vi "Write Data.vi"(8 "error in (no error)":errorcluster, 9 "Publication Time":timestamp, 10 "Value":variant, 11 "TerminalVisibilityBinding In":refnum<class "TerminalVisibilityBinding.lvclass">) -> (0 "error out":errorcluster, 3 "TerminalVisibilityBinding Out":refnum<class "TerminalVisibilityBinding.lvclass">)   [LabVIEW 2020, in "TerminalVisibilityBinding.lvclass"]
doc: "<License>\nCopyright © 2017 Composed Systems, LLC | All rights reserved\nwww.composed.io\n\nAuthor: Ethan Stern <ethan.stern@composed.io>\n\nThis software is provided \"AS IS\" WITHOUT WARRANTIES, either express or implied, AND IS FOR EDUCATIONAL PURPOSES ONLY.\n</License>"
uses:
  <vilib>/gpm_packages/@cs/transport/Source/Concrete/TerminalVisibilityBinding/TerminalVisibilityBinding.lvclass
  C:/Program Files/National Instruments/LabVIEW 2020/vi.lib/gpm_packages/@cs/transport/Source/Concrete/TerminalPropertyBinding/TerminalPropertyBinding.lvclass
  <vilib>/gpm_packages/@cs/transport/Source/Concrete/TerminalPropertyBinding/TerminalPropertyBinding.lvclass/TerminalPropertyBinding.ctl
  <vilib>/gpm_packages/@cs/transport/Source/Concrete/TerminalVisibilityBinding/TerminalVisibilityBinding.lvclass/TerminalVisibilityBinding.ctl
  <vilib>/Utility/error.llb/Error Cluster From Error Code.vi
  <vilib>/ErrorRing/Error Ring.xnode
  <vilib>/gpm_packages/@cs/transport/Source/Concrete/TerminalPropertyBinding/TerminalPropertyBinding.lvclass
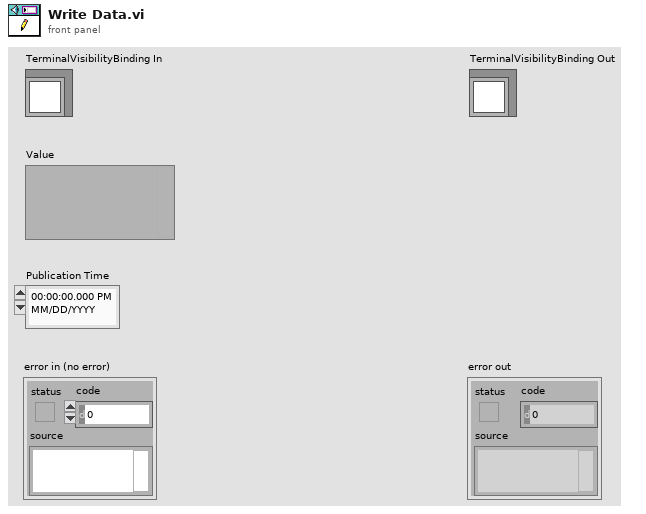
[diagram p1: front panel]
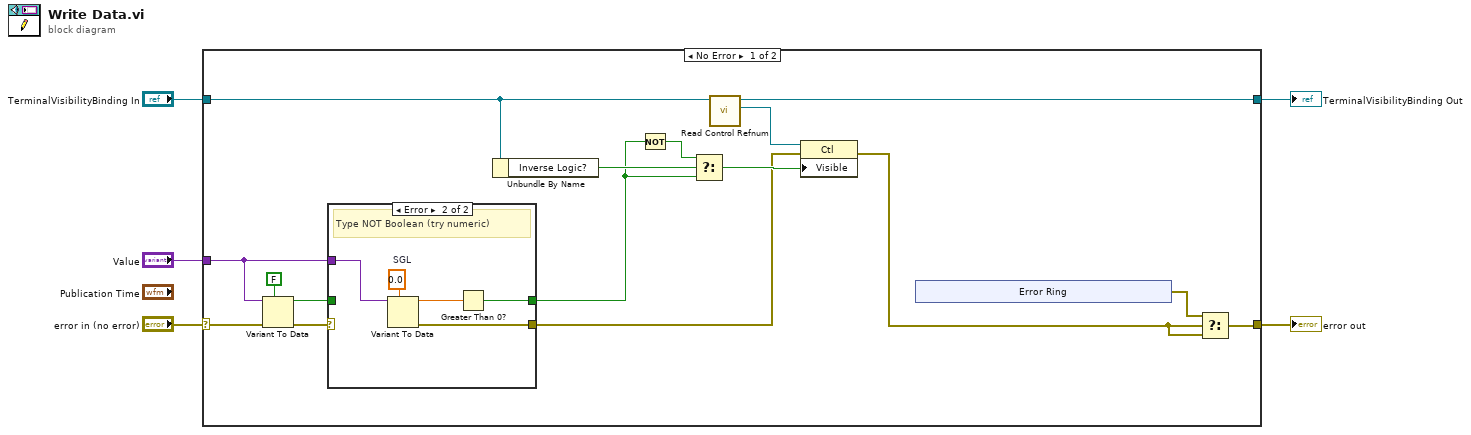
[diagram p0: block diagram]
diagram:
  n1 = case shown="No Error" "error in (no error)" {
    selector: "error in (no error)" -> [w10 w35]
    tunnel: "TerminalVisibilityBinding In" -> [w21 w34]
    tunnel: "Value" -> [w13 _]
    tunnel: [w12 w34] -> w2
    tunnel: [w6 w35] -> w1
    frame No Error {
      n2 = Variant To Data(error in=w10, type=FALSE, Variant=w13) -> (data=w16:bool, error out=w14:errorcluster)
      n3 = case shown="Error" w14 {
        selector: w14 -> [w27 _]
        tunnel: w16 -> [w28 _]
        tunnel: [w28 w31] -> w15
        tunnel: w13 -> [_ w30]
        tunnel: [w27 w29] -> w9
        frame No Error {
          # "Type = Boolean (OK)"
        }
        frame Error {
          w33 = sgl 0.0  # SGL
          # "Type NOT Boolean (try numeric)"
          n4 = Variant To Data(type=w33, Variant=w30) -> (data=w32:sgl, error out=w29:errorcluster)  [unwired: 1 in]
          n5 = Greater Than 0?(x=w32) -> (x > 0?=w31:bool)
        }
      }
      n6 = Unbundle By Name(w21) -> ("Inverse Logic?"=w19:bool)
      n7 = Not(x=w15) -> (.not. x?=w17:bool)
      n8 = Select(t=w17, s=w19, f=w15) -> (s? t:f=w18:bool)
      n9 = call <vilib>:"Read Control Refnum.vi"("TerminalReferenceBinding in"=w21) -> ("Ctl Refnum"=w11:refnum<vi>, "TerminalReferenceBinding out"=w12:refnum<class "TerminalVisibilityBinding.lvclass">)  [unwired: 9 in]
      n10 = property class="Ctl"(reference=w11, error in=w9, "Visible"=w18) -> (error out=w7:errorcluster)  [unwired: 1 out]
      n11 = xnode "Error Ring"() -> ("error out"=w8:errorcluster)
      n12 = Select(t=w8, s=w7, f=w7) -> (s? t:f=w6:errorcluster)
    }
    frame Error {
    }
  }
  "error out" <- w1
  "TerminalVisibilityBinding Out" <- w2
